vi "Read Trigger.vi"(8 "error in (no error)":errorcluster, 11 "VISA resource name":refnum<visa-resource-name>) -> (0 "error out":errorcluster, 2 "Trigger Activated":bool, 3 "VISA resource name out":refnum<visa-resource-name>)   [LabVIEW 2020, in "BDAQ-6104.lvlib"]
uses:
  <instrlib>/BDAQ-6104/BDAQ-6104.lvlib
  <vilib>/Instr/_visa.llb/VISA Flush IO Buffer Mask.ctl
panel:
  out "read buffer":string
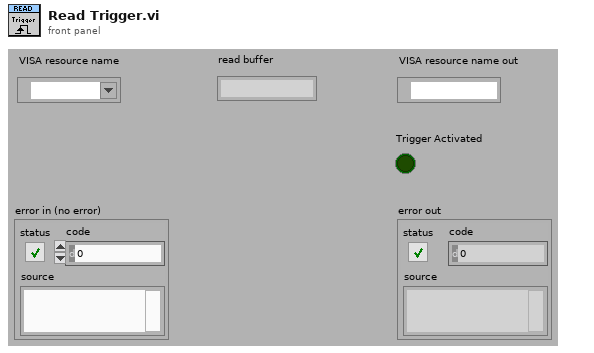
[diagram p1: front panel]
types:
  T1 = typedef "VISA Flush IO Buffer Mask.ctl" = u16
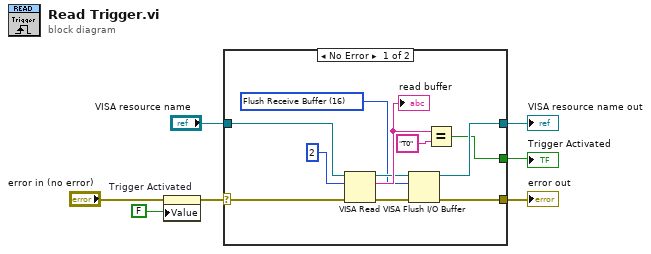
[diagram p0: block diagram]
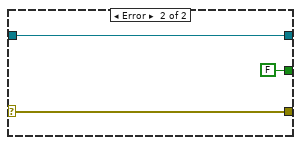
[diagram p2: hidden frame]
diagram:
  n1 = property on="Trigger Activated" class="Bool (strict)"(error in="error in (no error)", "Value"=FALSE ("Trigger Activated")) -> (error out=w2:errorcluster)  [unwired: 1 in, 1 out]
  n2 = case shown="No Error" w2 {
    selector: w2 -> [w10 w20]
    tunnel: "VISA resource name" -> [w12 w21]
    tunnel: [w11 w21] -> w6
    tunnel: [w9 w20] -> w5
    tunnel: [w8 FALSE] -> w4
    frame No Error {
      w13 = T1 16 items=["Flush Receive Buffer"=16, "Write Transmit Buffer to Device"=32, "Flush Receive Buffer (No I/O)"=64, "Flush Transmit Buffer"=128] ("Mask")
      n3 = VISA Read(VISA resource name=w12, byte count=u32 2, error in (no error)=w10) -> (VISA resource name out=w14:refnum<visa-resource-name>, read buffer=w17:string, error out=w15:errorcluster)  [unwired: 1 out]
      "read buffer" <- w17
      n4 = VISA Flush I/O Buffer(VISA resource name=w14, mask (16)=w13, error in (no error)=w15) -> (VISA resource name out=w11:refnum<visa-resource-name>, error out=w9:errorcluster)
      n5 = Equal?(x=w17, y="T0") -> (x = y?=w8:bool)
    }
    frame Error {
    }
  }
  "VISA resource name out" <- w6
  "error out" <- w5
  "Trigger Activated" <- w4
